vi "Configure Measurement Manual Range.vi"(8 "error in (no error)":errorcluster, 9 "Manual Range (1.0)":dbl=0.1, 10 "Function (0: Volts)":u16(ring) items=["Volts", "Current", "Resistance", "Digitize Volts", "Digitize Current"], 11 "VISA resource name":refnum<visa-resource-name>="USB0::0x05E6::0x2461::04090176::INSTR") -> (0 "error out":errorcluster, 3 "VISA resource name out":refnum<visa-resource-name>="USB0::0x05E6::0x2461::04090176::INSTR")   [LabVIEW 2022 SP3, in "Keithley 2450.lvlib"]
doc: "This VI sets the positive full-scale value of the measurement range for measurements of the selected function.\n\n<B>The Digitize Voltage and Digitize Current functions are only valid on the 2461</B>"
uses:
  Keithley 2450.lvlib
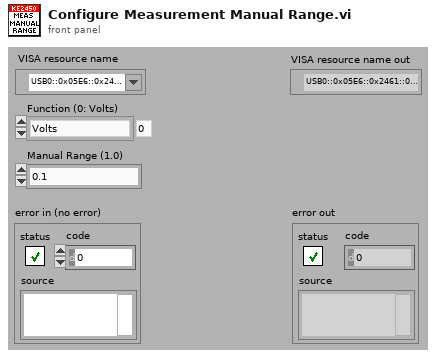
[diagram p1: front panel]
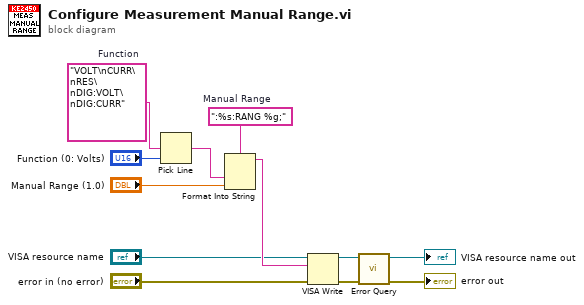
[diagram p0: block diagram]
diagram:
  w7 = "VOLT\nCURR\nRES\nDIG:VOLT\nDIG:CURR"  # Function
  w9 = ":%s:RANG %g;"  # Manual Range
  n1 = Pick Line(multi-line string=w7, line index="Function (0: Volts)") -> (output string=w5:string)  [unwired: 1 out]
  n2 = Format Into String(format string=w9, w5, "Manual Range (1.0)") -> (resulting string=w10:string)  [unwired: 2 in, 1 out]
  n3 = VISA Write(VISA resource name="VISA resource name", write buffer=w10, error in (no error)="error in (no error)") -> (VISA resource name out=w4:refnum<visa-resource-name>, error out=w3:errorcluster)  [unwired: 1 out]
  n4 = call "Error Query.vi"("error in (no error)"=w3, "VISA resource name"=w4) -> ("error out"=→"error out":errorcluster, "VISA resource name out"=→"VISA resource name out":refnum<visa-resource-name>)  [unwired: 8 out]
